vi "Controller - State Entry.vi"(8 "error in (no error)":errorcluster, 11 "View Model":T1) -> (0 "error out":errorcluster, 3 "View Model":T1)   [LabVIEW 2017]
doc: "Initializes state information at beginning of transition."
uses:
  View Model/Controls/View Model.ctl
  View Model/Controls/Shared Model.ctl
  Error Handler/Controls/Error Model.ctl
  Error Handler/Controls/Error Data.ctl
  Error Handler/Controls/Error Level.ctl
  Configuration/Controls/Config Model.ctl
  Configuration/Controls/Config Record.ctl
  Configuration/Controls/Config Data.ctl
  Configuration/Controls/Config Command.ctl
  Controls/Controler Model.ctl
  Views/Vehicle Position View/Controls/Vehicle - Station Slider.ctl
  Views/Entry Console View/Controls/Entry Console - Wash Steps.ctl
  Controls/Controller - Event.ctl
  Controls/Controller - Commands.ctl
  Controls/Controller - Overhead.ctl
  Controls/Controller - States.ctl
  Controls/Controller - Wash Step.ctl
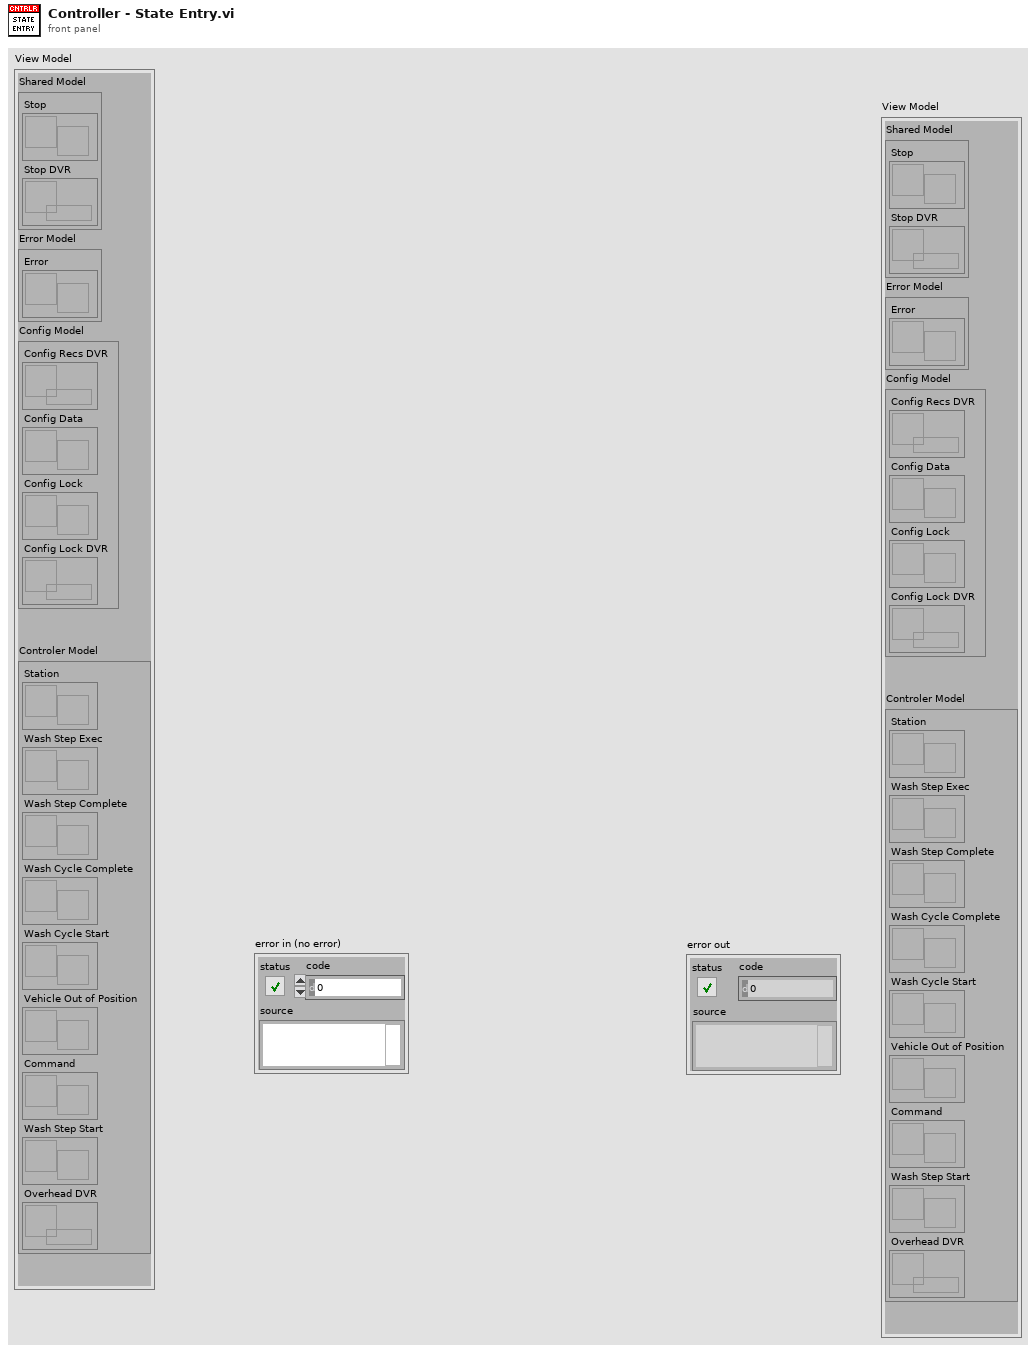
[diagram p1: front panel]
types:
  T1 = typedef "View Model.ctl" = cluster{"Shared Model":T2, "Error Model":T3, "Config Model":T4, "Controler Model":T5}
  T2 = typedef "Shared Model.ctl" = cluster{"Stop":refnum<user-event>, "Stop DVR":refnum<data-value>}
  T3 = typedef "Error Model.ctl" = cluster{"Error":refnum<user-event>}
  T4 = typedef "Config Model.ctl" = cluster{"Config Recs DVR":refnum<data-value>, "Config Data":refnum<user-event>, "Config Lock":refnum<user-event>, "Config Lock DVR":refnum<data-value>}
  T5 = typedef "Controler Model.ctl" = cluster{"Station":refnum<user-event>, "Wash Step Exec":refnum<user-event>, "Wash Step Complete":refnum<user-event>, "Wash Cycle Complete":refnum<user-event>, "Wash Cycle Start":refnum<user-event>, "Vehicle Out of Position":refnum<user-event>, "Command":refnum<user-event>, "Wash Step Start":refnum<user-event>, "Overhead DVR":refnum<data-value>}
  T6 = typedef "Controller - States.ctl" = enum16{"Initial", "Wait for Start", "Wash Cycle Start", "Wait for Vehicle Position", "Wash Step Start", "Wash Step Execute", "Wash Step Complete", "Wash Cycle Complete", "Wash Exit", "Wash Abort/Terminate"}
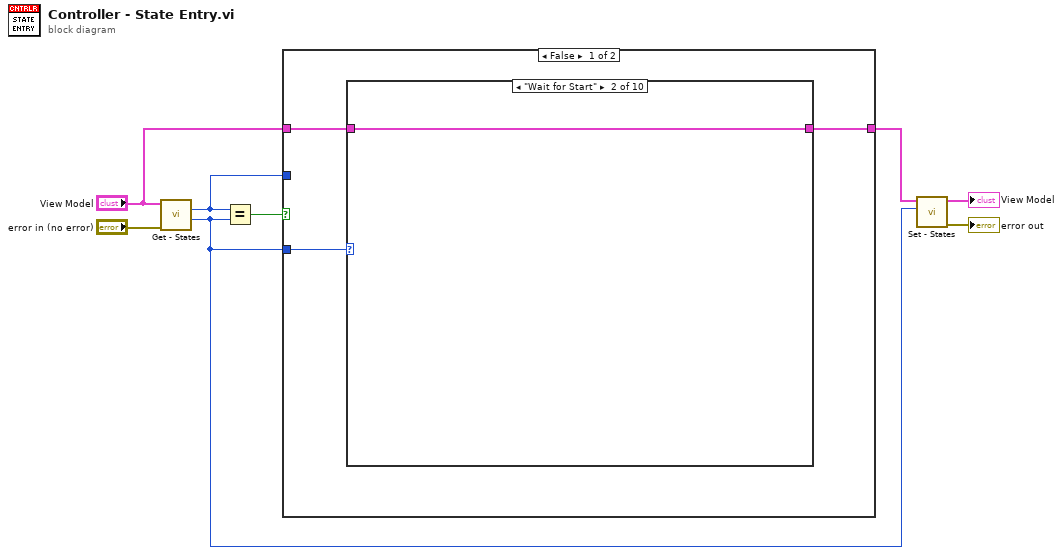
[diagram p0: block diagram]
diagram:
  n1 = call "Get - States.vi"("error in (no error)"="error in (no error)", "View Model"="View Model") -> ("Next State"=w2:T6, "Current State"=w6:T6)  [unwired: 6 in, 2 out]
  n2 = Equal?(x=w6, y=w2) -> (x = y?=w7:bool)
  n3 = case shown="False" w7 {
    tunnel: w2 -> [w11 _]
    tunnel: w6 -> [_ _]
    tunnel: "View Model" -> [w10 w22]
    tunnel: [w9 w22] -> w4
    frame False {
      n4 = case shown="\"Wait for Start\"" w11 {
        tunnel: w10 -> [w12 w13 w14 w15 w16 w17 w18 w19 w20 w21]
        tunnel: [w12 w13 w14 w15 w16 w17 w18 w19 w20 w21] -> w9
        frame "Initial", Default {
        }
        frame "Wait for Start" {
        }
        frame "Wash Cycle Start" {
        }
        frame "Wait for Vehicle Position" {
        }
        frame "Wash Step Start" {
        }
        frame "Wash Step Execute" {
        }
        frame "Wash Step Complete" {
        }
        frame "Wash Cycle Complete" {
        }
        frame "Wash Exit" {
        }
        frame "Wash Abort/Terminate" {
        }
      }
    }
    frame True {
    }
  }
  n5 = call "Set - States.vi"("Current State"=w2, "View Model"=w4) -> ("error out"=→"error out":errorcluster, "View Model"=→"View Model":T1)  [unwired: 8 in]
